vi "DAQ.Create AI Tasks.vi"(8 "error in":errorcluster, 11 "Instrument.DAQ":refnum<class "Instrument.DAQ.lvclass">) -> (0 "error out":errorcluster, 3 "Instrument.DAQ":refnum<class "Instrument.DAQ.lvclass">)   [LabVIEW 2019, in "Instrument.DAQ.lvclass"]
uses:
  Instrument.DAQ.lvclass
  Instrument.DAQ.lvclass/Instrument.DAQ.ctl
  <vilib>/DAQmx/create/channels.llb/DAQmx Create Channel (AI-Voltage-Basic).vi
  <resource>/objmgr/daqmx.rc
panel:
  out "Current Size":i32
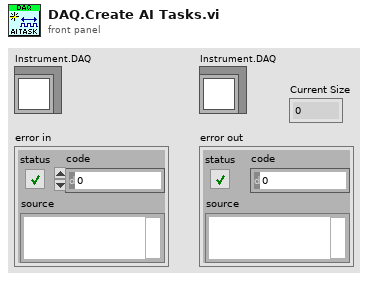
[diagram p1: front panel]
types:
  T1 = typedef "Instrument.DAQ.lvclass/DAQ.Config.AI--Cluster--Array.ctl" = T2[]
  T2 = typedef "Instrument.DAQ.lvclass/DAQ.Config.AI--Cluster.ctl" = cluster{"Channels":tag, "Coupling":T3, "Range":T4, "input terminal configuration":i32, "Type":T5}
  T3 = typedef "Instrument.DAQ.lvclass/DAQ.Config.AI.Coupling--enum.ctl" = u16
  T4 = typedef "Instrument.DAQ.lvclass/DAQ.Config.AI.Range--enum.ctl" = enum16{"±0.316", "±1.00", "±3.16", "±10.0", "±31.6", "±42.4"}
  T5 = typedef "Instrument.DAQ.lvclass/DAQ.Type--enum.ctl" = enum16{"None", "USB 4431", "PXI 446x"}
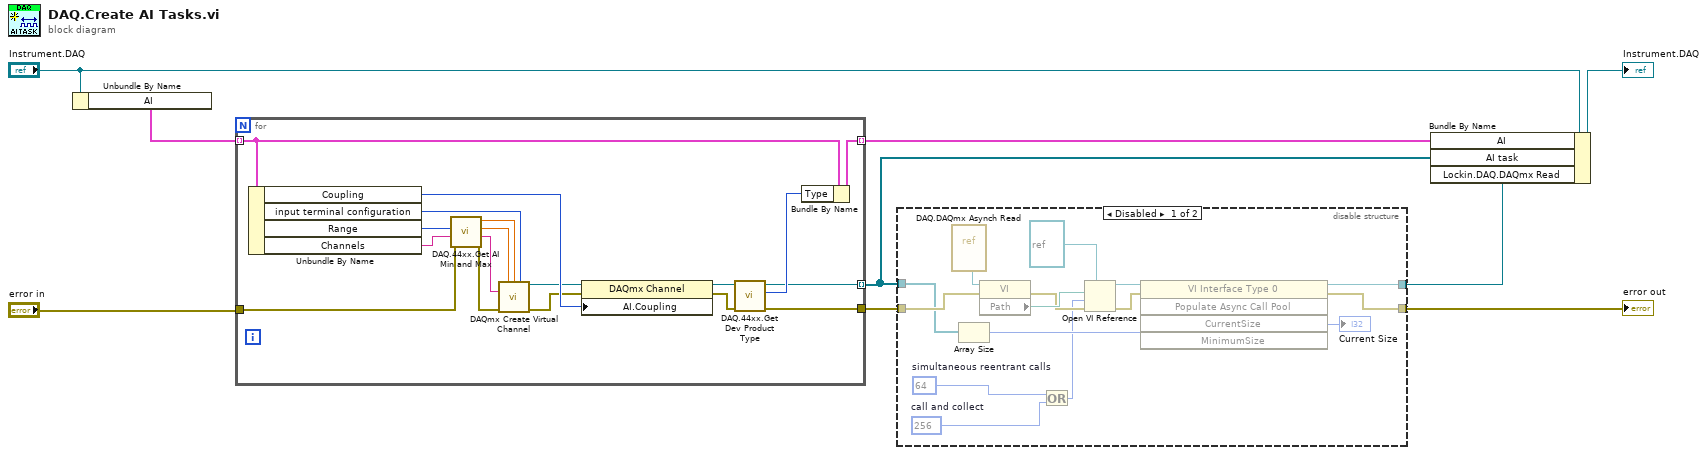
[diagram p0: block diagram]
diagram:
  n1 = Unbundle By Name("Instrument.DAQ") -> ("AI"=w5:T1)
  n2 = for {
    tunnel: [w21] -> w7 mode=indexing
    tunnel: w5 -> [w22] mode=indexing
    tunnel: "error in" -> [w10]
    tunnel: [w15] -> w4
    tunnel: [w16] -> w1 mode=indexing
    n3 = Unbundle By Name(w22) -> ("Coupling"=w26:T3, "input terminal configuration"=w27:i32, "Range"=w14:T4, "Channels"=w12:tag)
    n4 = call "DAQ.44xx.Get AI Min and Max.vi"("error in (no error)"=w10, "AI.channels"=w12, "AI.Range"=w14) -> ("error out"=w11:errorcluster, "AI.channels out"=w13:tag, "AI.Max"=w24:dbl, "AI.Min"=w25:dbl)  [unwired: 5 in]
    n5 = call-poly <vilib>:"DAQmx Create Virtual Channel.vi"("maximum value"=w24, "minimum value"=w25, "input terminal configuration"=w27, "physical channels"=w13, "error in"=w11) -> ("task out"=w20:refnum<k21>, "error out"=w23:errorcluster)  [unwired: 9 in]
    n6 = property class="DAQmx Channel"(reference=w20, error in=w23, "AI.Coupling"=w26) -> (reference out=w19:refnum<k21>, error out=w18:errorcluster)
    n7 = call "DAQ.44xx.Get Dev Product Type.vi"("error in (no error)"=w18, "Refnum in"=w19) -> ("error out"=w15:errorcluster, "DAQ Type"=w17:T5, "Refnum out"=w16:refnum<k21>)  [unwired: 6 in, 1 out]
    n8 = Bundle By Name(cluster=w22, "Type"=w17) -> (w21:T2)
  }
  n9 = disable-structure shown="Disabled" {
    disable-tunnel: w4 -> [w37 w43]
    disable-tunnel: [w36 w43] -> w3
    disable-tunnel: [w35 _] -> w2
    disable-tunnel: w1 -> [w32 _]
    frame Disabled {
      w30 = 64  # simultaneous reentrant calls
      w28 = 256  # call and collect
      n10 = vi-ref "DAQ.DAQmx Asynch Read.vi"() -> (w33:refnum<vi>)
      n11 = Array Size(array=w32) -> (size(s)=w31:i32)
      n12 = property class="VI"(reference=w33, error in=w37) -> (error out=w41:errorcluster, "Path"=w42:path)  [unwired: 1 out]
      n13 = Or(x=w30, y=w28) -> (x .or. y?=w29:i32)
      n14 = Open VI Reference(type specifier VI Refnum (for type only)=refnum<vi> refnum, vi path=w42, options=w29, error in (no error)=w41) -> (vi reference=w39:refnum<vi>, error out=w38:errorcluster)  [unwired: 2 in]
      n15 = invoke class="VI Interface Type 0" method="Populate Async Call Pool"(reference=w39, error in=w38, "MinimumSize"=w31) -> (reference out=w35:refnum<vi>, error out=w36:errorcluster, "CurrentSize"=→"Current Size":i32)  [unwired: 2 in, 2 out]
    }
    frame Enabled {
    }
  }
  "error out" <- w3
  n16 = Bundle By Name(cluster="Instrument.DAQ", "AI"=w7, "AI task"=w1, "Lockin.DAQ.DAQmx Read"=w2) -> (→"Instrument.DAQ":refnum<class "Instrument.DAQ.lvclass">)
